vi "Read Available Data Names.vi"(8 "error in (no error)":errorcluster, 11 "ControlDragOverMsg In":refnum<class "ControlDragOverMsg.lvclass">) -> (0 "error out":errorcluster, 2 "Available Data Names":string[](array[string]), 3 "ControlDragOverMsg Out":refnum<class "ControlDragOverMsg.lvclass">)   [LabVIEW 2019, in "ActorEvents.lvlib" / "ControlDragOverMsg.lvclass"]
uses:
  <vilib>/gpm_packages/@cs/mva-viewable/Source/ActorEvents/IEventAggregator Messages/ControlDragOverMsg/ControlDragOverMsg.lvclass
  <vilib>/gpm_packages/@cs/mva-viewable/Source/ActorEvents/IEventAggregator Messages/ControlDragOverMsg/ControlDragOverMsg.lvclass/ControlDragOverMsg.ctl
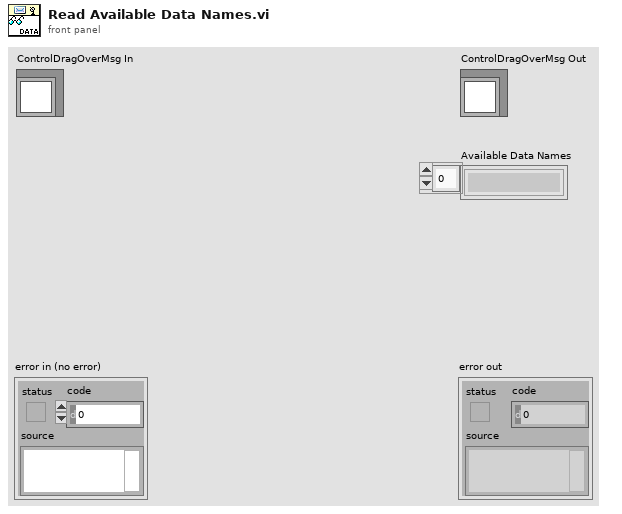
[diagram p1: front panel]
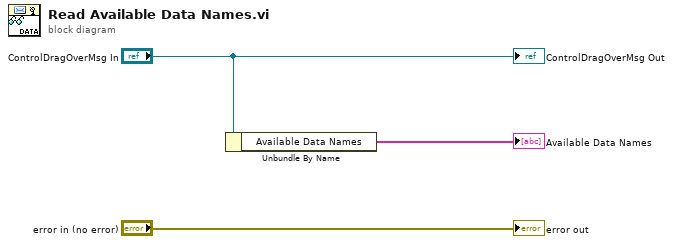
[diagram p0: block diagram]
diagram:
  n1 = Unbundle By Name("ControlDragOverMsg In") -> ("Available Data Names"=→"Available Data Names":string[])
  "error out" <- "error in (no error)"
  "ControlDragOverMsg Out" <- "ControlDragOverMsg In"
